vi "Measure Temperature Board.vi"(0 "COM Port in":refnum<visa-resource-name>, 1 "error in":errorcluster) -> (2 "COM Port out":refnum<visa-resource-name>, 3 "temperature":dbl format="%#.1f", 4 "OK":bool, 5 "error out":errorcluster)   [LabVIEW 2013]
doc: "This command measures the actual temperature at the PCB inside the laser controller."
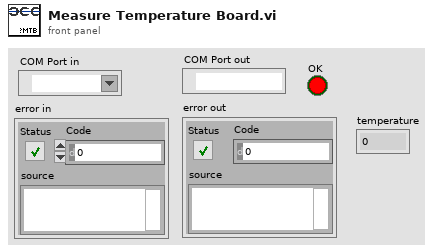
[diagram p1: front panel]
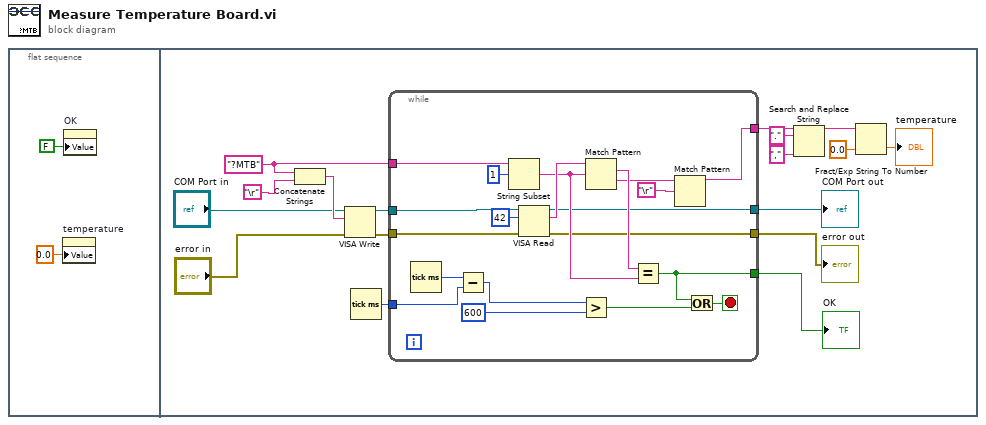
[diagram p0: block diagram]
diagram:
  n1 = flat-sequence {
    frame #0 {
      n2 = property on="temperature" class="DigWert (strikt)"("Value"=0.0 ("temperature")) -> ()  [unwired: 2 in, 2 out]
      n3 = property on="OK" class="Bool. (strikt)"("Value"=FALSE ("OK")) -> ()  [unwired: 2 in, 2 out]
    }
    frame #1 {
      w8 = "?MTB" ("Schreibpuffer")
      n4 = Concatenate Strings(w8, "\r") -> (w14:string)
      n5 = VISA Write(VISA resource name="COM Port in", write buffer=w14, error in (no error)="error in") -> (VISA resource name out=w10:refnum<visa-resource-name>, error out=w9:errorcluster)  [unwired: 1 out]
      n6 = Tick Count (ms)() -> (millisecond timer value=w3:u32)
      n7 = while {
        tunnel: [w34] -> w19
        tunnel: [w33] -> w18
        tunnel: [w32] -> w7
        tunnel: [w28] -> w17
        tunnel: w10 -> [w21]
        tunnel: w9 -> [w30]
        tunnel: w8 -> [w29]
        tunnel: w3 -> [w25]
        stop <- w27 stop-if-true
        n8 = Tick Count (ms)() -> (millisecond timer value=w26:u32)
        n9 = Subtract(x=w26, y=w25) -> (x-y=w24:u32)
        n10 = String Subset(string=w29, offset (0)=1 ("Offset (0)")) -> (substring=w35:string)  [unwired: 1 in]
        n11 = VISA Read(VISA resource name=w21, byte count=u32 42 ("Byte-Anzahl"), error in (no error)=w30) -> (VISA resource name out=w34:refnum<visa-resource-name>, read buffer=w38:string, error out=w33:errorcluster)  [unwired: 1 out]
        n12 = Greater?(x=w24, y=u32 600) -> (0:w22:bool)
        n13 = Match Pattern(string=w38, regular expression=w35) -> (match substring=w37:string, after substring=w31:string)  [unwired: 1 in, 2 out]
        n14 = Equal?(x=w37, y=w35) -> (x = y?=w28:bool)
        n15 = Match Pattern(string=w31, regular expression="\r") -> (before substring=w32:string)  [unwired: 1 in, 3 out]
        n16 = Or(x=w28, y=w22) -> (x .or. y?=w27:bool)
      }
      "COM Port out" <- w19
      "error out" <- w18
      "OK" <- w17
      n17 = Search and Replace String(input string=w7, search string="." ("Such-String"), replace string="," ("String ersetzen(\"\")")) -> (result string=w6:string)  [unwired: 5 in, 3 out]
      n18 = Fract/Exp String To Number(string=w6, default (0 dbl)=0.0 ("Standard (0 DBL)")) -> (number=→"temperature":dbl)  [unwired: 2 in, 1 out]
    }
  }
